vi "T89.vi"() -> ()   [LabVIEW 2024]
uses:
  <vilib>/Instr/_visa.llb/VISA Configure Serial Port (Instr).vi
panel:
  in  "Bleu":u8(slide) scale=0.0..255.0
  in  "Vert":u8(slide) scale=0.0..255.0
  in  "Ruge":u8(slide) scale=0.0..255.0
  in  "Stop":bool
  out "LED RGB":bool[](array[boolean])
  out "Bleu":u8
  out "Vert":u8
  out "Ruge":u8
  out "Envoye:":string
  out "Reponse:":string
  in  "VISA":refnum<visa-resource-name>
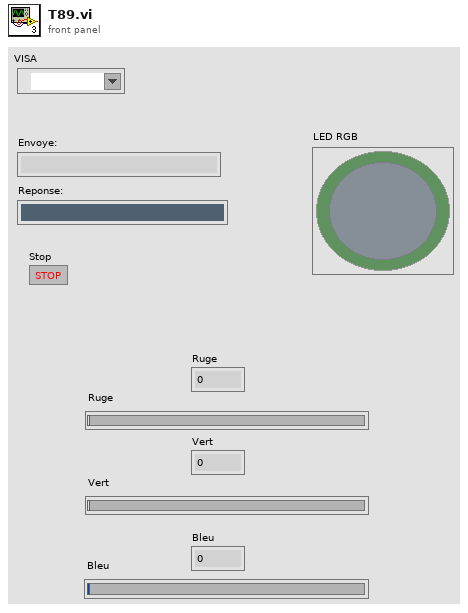
[diagram p1: front panel]
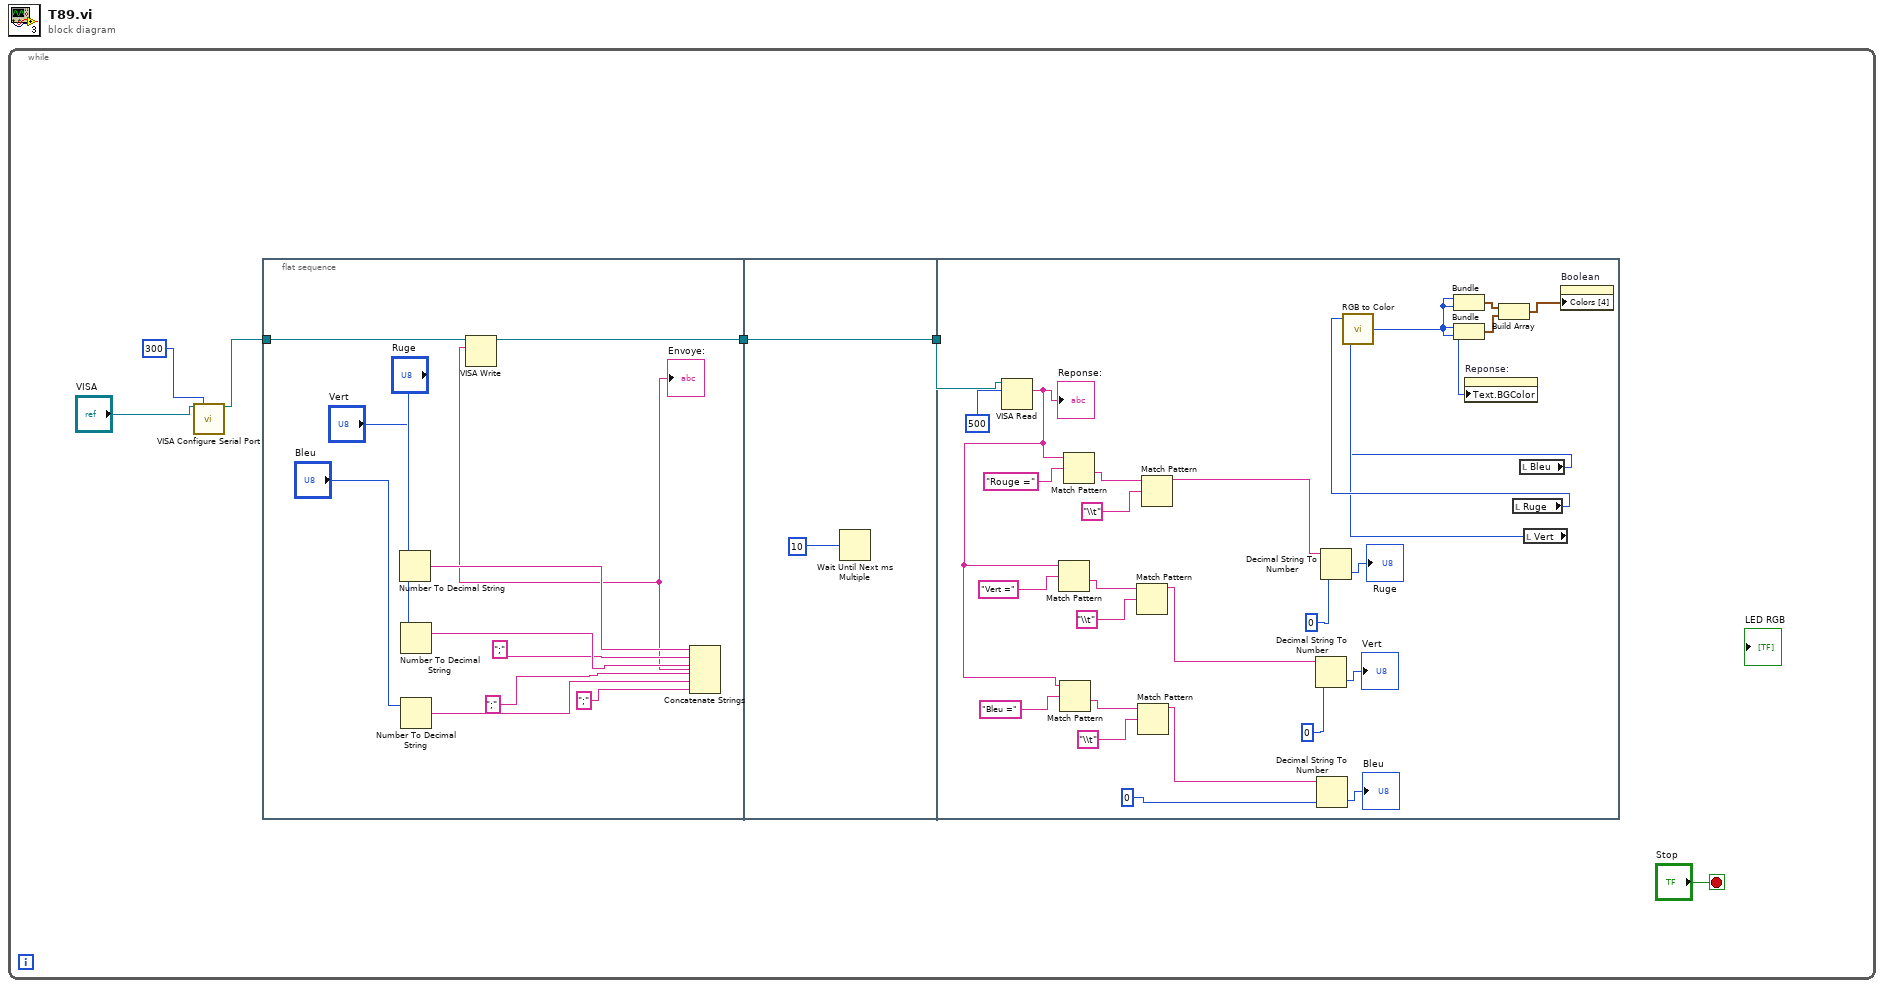
[diagram p0: block diagram]
diagram:
  n1 = while {
    stop <- "Stop" stop-if-true
    n2 = call-poly "VISA Configure Serial Port"("VISA resource name"="VISA", "timeout (10sec)"=300) -> ("VISA resource name out"=w2:refnum<visa-resource-name>)  [unwired: 12 in, 1 out]
    n3 = flat-sequence {
      tunnel: w2 -> [w18]
      tunnel: [w17] -> w6
      tunnel: w6 -> [w19]
      tunnel: [w19] -> w5
      tunnel: w5 -> [w48]
      frame #0 {
        n4 = Number To Decimal String(number="Ruge") -> (decimal integer string=w14:string)  [unwired: 1 in]
        n5 = Number To Decimal String(number="Vert") -> (decimal integer string=w16:string)  [unwired: 1 in]
        n6 = Number To Decimal String(number="Bleu") -> (decimal integer string=w15:string)  [unwired: 1 in]
        n7 = Concatenate Strings(w14, ";", w16, ";", w15, ";") -> (w10:string)
        "Envoye:" <- w10
        n8 = VISA Write(VISA resource name=w18, write buffer=w10) -> (VISA resource name out=w17:refnum<visa-resource-name>)  [unwired: 1 in, 2 out]
      }
      frame #1 {
        n9 = Wait Until Next ms Multiple(millisecond multiple=10) -> ()  [unwired: 1 out]
      }
      frame #2 {
        n10 = VISA Read(VISA resource name=w48, byte count=500) -> (read buffer=w31:string)  [unwired: 1 in, 3 out]
        "Reponse:" <- w31
        n11 = Match Pattern(string=w31, regular expression="Vert =") -> (after substring=w38:string)  [unwired: 1 in, 3 out]
        n12 = Match Pattern(string=w31, regular expression="Bleu =") -> (after substring=w35:string)  [unwired: 1 in, 3 out]
        n13 = Match Pattern(string=w31, regular expression="Rouge =") -> (after substring=w45:string)  [unwired: 1 in, 3 out]
        n14 = Match Pattern(string=w38, regular expression="\\t") -> (before substring=w39:string)  [unwired: 1 in, 3 out]
        n15 = Match Pattern(string=w35, regular expression="\\t") -> (before substring=w34:string)  [unwired: 1 in, 3 out]
        n16 = Match Pattern(string=w45, regular expression="\\t") -> (before substring=w44:string)  [unwired: 1 in, 3 out]
        n17 = Decimal String To Number(string=w39, default (0L)=0) -> (number=→"Vert":i32)  [unwired: 1 in, 1 out]
        n18 = Decimal String To Number(string=w34, default (0L)=0) -> (number=→"Bleu":i32)  [unwired: 1 in, 1 out]
        n19 = Decimal String To Number(string=w44, default (0L)=0) -> (number=→"Ruge":i32)  [unwired: 1 in, 1 out]
        n20 = local read "Ruge"() -> (w23:u8)
        n21 = local read "Bleu"() -> (w21:u8)
        n22 = local read "Vert"() -> (w22:u8)
        n23 = call <vilib>:"RGB to Color.vi"("B"=w21, "G"=w22, "R"=w23) -> ("Color"=w27:u32)
        n24 = Bundle("Color"=w27, "Color"=w27) -> (w26:cluster{"Color":u32, "Color":u32})  [unwired: 1 in]
        n25 = Bundle("Color"=w27, "Color"=w27) -> (w25:cluster{"Color":u32, "Color":u32})  [unwired: 1 in]
        n26 = property on="Reponse:" class="Str"("Text.BGColor"=w27) -> ()  [unwired: 2 in, 2 out]
        n27 = Build Array(w26, w25) -> (w24:cluster{"Color":u32, "Color":u32}[])
        n28 = property on="Boolean" class="Bool (strict)"("Colors [4]"=w24) -> ()  [unwired: 2 in, 2 out]
      }
    }
  }
